vi "substreepbocht.vi"(4 "tijdsinterval 8":dbl, 5 "tijdsinterval 6":dbl, 6 "tijdsinterval 7":dbl, 7 "tijdsinterval in":dbl, 9 "tijdsinterval 5":dbl, 10 "tijdsinterval 3":dbl, 11 "tijdsinterval 4":dbl) -> ()   [LabVIEW 2019]
uses:
  <vilib>/myRIO/Common/Instrument Driver Framework/Utilities/typedefs/Analog Scaling Constants.ctl
  <vilib>/myRIO/Common/Instrument Driver Framework/Utilities/typedefs/Analog Scaling Constants List.ctl
  <vilib>/myRIO/Common/Instrument Driver Framework/myRIO v1.0/AO/typedefs/AO Channels Enum.ctl
  <vilib>/myRIO/Common/Instrument Driver Framework/myRIO v1.0/AO/typedefs/AO Channels List.ctl
  <vilib>/myRIO/Common/Instrument Driver Framework/Utilities/typedefs/Generic FPGA Reference.ctl
  <vilib>/myRIO/Common/Instrument Driver Framework/Utilities/typedefs/myRIO v1.0 Reference.ctl
  <vilib>/myRIO/Common/Instrument Driver Framework/Utilities/typedefs/Hardware Version Enum.ctl
  <vilib>/myRIO/Common/Instrument Driver Framework/Utilities/typedefs/myRIO Generic Hardware Reference.ctl
  <vilib>/myRIO/Instrument Drivers/Onboard IO/AO/typedefs/AO Reference.ctl
  <vilib>/myRIO/Instrument Drivers/Onboard IO/AO/AO.lvlib
  <vilib>/myRIO/Instrument Drivers/Onboard IO/AO/vis/Write.vi
  <vilib>/userDefined/High Color/nirio_resource_hc.ctl
  <vilib>/myRIO/Common/Instrument Driver Framework/myRIO v1.0/AO/vis/myRIO v1.1 Open AO.vi
  <vilib>/myRIO/Instrument Drivers/Onboard IO/AO/vis/myRIO AO Open.xnode
  <vilib>/myRIO/Common/Instrument Driver Framework/Utilities/vis/Is FPGA Ref Available.vi
  <vilib>/myRIO/Express VI/Onboard IO/AO/AO Express VI.xnode
  Global.vi
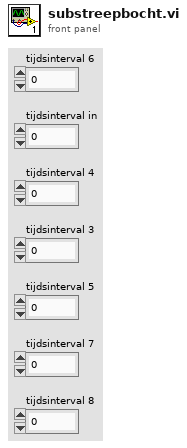
[diagram p1: front panel]
types:
  T1 = typedef "AO.lvlib/AO Reference.ctl" = cluster{"myRIO Reference":T2, "AO Channel List":T6, "AO Scaling Constant List":T8}
  T2 = typedef "myRIO Generic Hardware Reference.ctl" = cluster{"myRIO Model":T3, "myRIO Hardware Reference":T4}
  T3 = typedef "Hardware Version Enum.ctl" = enum16{"Unknown", "myRIO-1900", "myRIO-1950", "roboRIO", "NI ELVIS RIO CM", "ELVIS III"}
  T4 = typedef "myRIO v1.0 Reference.ctl" = cluster{"Generic FPGA Reference":T5, "Allow multiple opens":bool}
  T5 = typedef "Generic FPGA Reference.ctl" = refnum<k20>
  T6 = typedef "AO Channels List.ctl" = T7[]
  T7 = typedef "AO Channels Enum.ctl" = enum16{"Not Connected", "AudioOut/Left", "AudioOut/Right", "C/AO0", "C/AO1", "A/AO0", "A/AO1", "B/AO0", "B/AO1"}
  T8 = typedef "Analog Scaling Constants List.ctl" = T9[]
  T9 = typedef "Analog Scaling Constants.ctl" = cluster{"LSB Weight (Volts)":dbl, "Offset (Volts)":dbl, "Signed?":bool}
  T10 = typedef "nirio_resource_hc.ctl" = tag
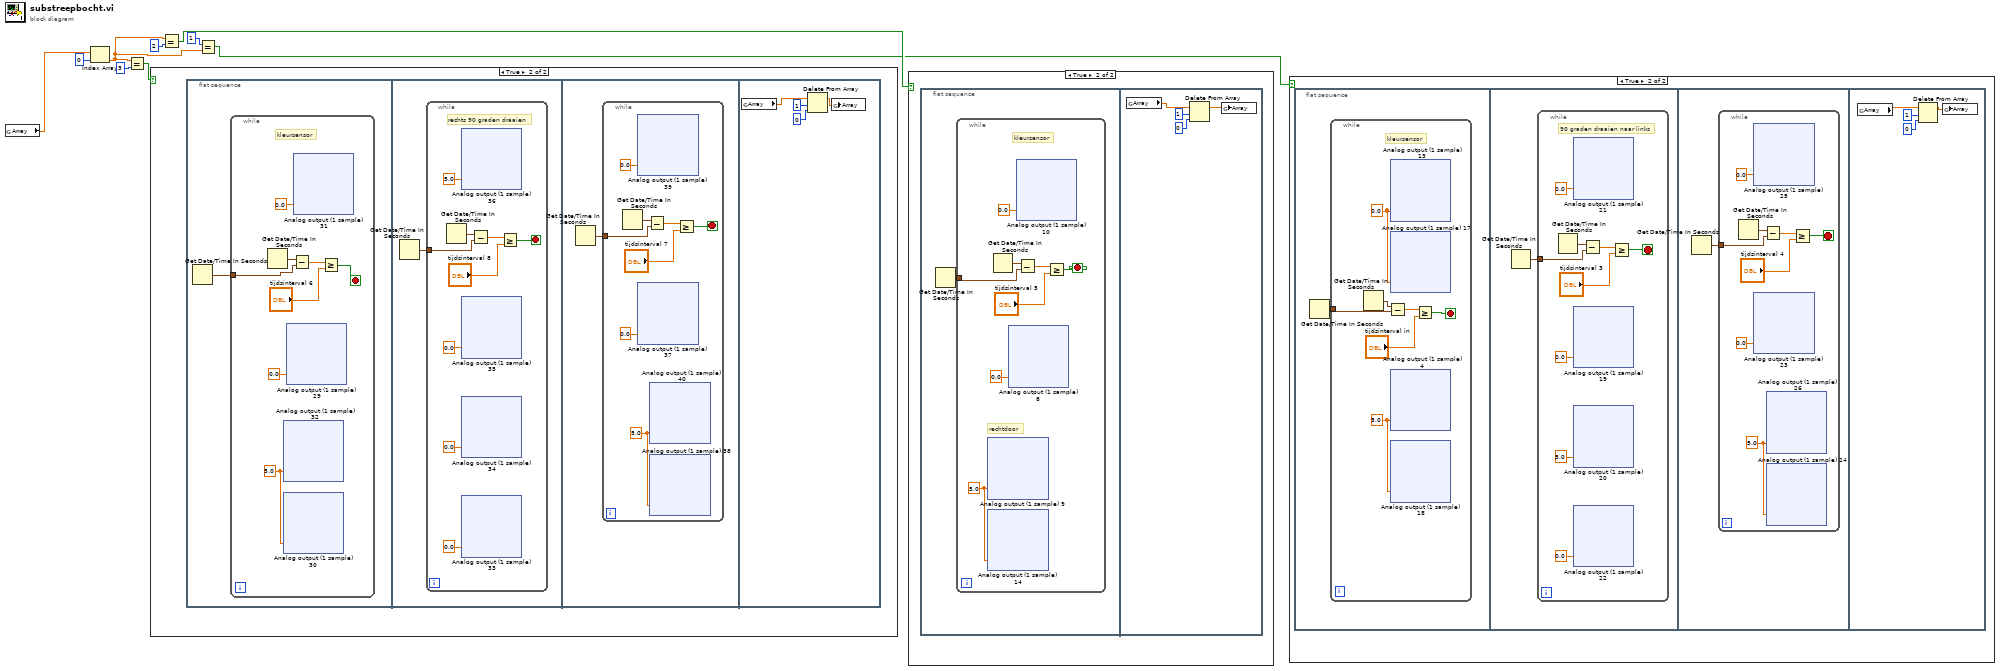
[diagram p0: block diagram]
diagram:
  n1 = global read "Global.vi" "Array"() -> (w9:dbl[])
  n2 = Index Array(array=w9, index=0) -> (element=w5:dbl)
  n3 = Equal?(x=w5, y=3) -> (x = y?=w3:bool)
  n4 = case shown="True" w3 {
    frame False {
    }
    frame True {
      n5 = flat-sequence {
        frame #0 {
          n6 = Get Date/Time In Seconds() -> (seconds since 1Jan1904=w10:timestamp)
          n7 = while {
            tunnel: w10 -> [w15]
            stop <- w11 stop-if-true
            w13 = 5.0
            # "kleursensor"
            n8 = Get Date/Time In Seconds() -> (seconds since 1Jan1904=w18:timestamp)
            n9 = xnode "Analog output (1 sample) 32"("A/AO0 (Pin 2)"=w13) -> ()  [unwired: 1 in, 1 out]
            n10 = xnode "Analog output (1 sample) 30"("B/AO0 (Pin 2)"=w13) -> ()  [unwired: 1 in, 1 out]
            n11 = xnode "Analog output (1 sample) 29"("B/AO1 (Pin 4)"=0.0) -> ()  [unwired: 1 in, 1 out]
            n12 = Subtract(x=w18, y=w15) -> (x-y=w16:dbl)
            n13 = xnode "Analog output (1 sample) 31"("A/AO1 (Pin 4)"=0.0) -> ()  [unwired: 1 in, 1 out]
            n14 = Greater Or Equal?(x=w16, y="tijdsinterval 6") -> (x >= y?=w11:bool)
          }
        }
        frame #1 {
          n15 = Get Date/Time In Seconds() -> (seconds since 1Jan1904=w167:timestamp)
          n16 = while {
            tunnel: w167 -> [w169]
            stop <- w170 stop-if-true
            # "rechts 90 graden draaien"
            n17 = Get Date/Time In Seconds() -> (seconds since 1Jan1904=w173:timestamp)
            n18 = xnode "Analog output (1 sample) 36"("A/AO0 (Pin 2)"=5.0) -> ()  [unwired: 1 in, 1 out]
            n19 = xnode "Analog output (1 sample) 35"("A/AO1 (Pin 4)"=0.0) -> ()  [unwired: 1 in, 1 out]
            n20 = xnode "Analog output (1 sample) 34"("B/AO0 (Pin 2)"=0.0) -> ()  [unwired: 1 in, 1 out]
            n21 = xnode "Analog output (1 sample) 33"("B/AO1 (Pin 4)"=0.0) -> ()  [unwired: 1 in, 1 out]
            n22 = Subtract(x=w173, y=w169) -> (x-y=w171:dbl)
            n23 = Greater Or Equal?(x=w171, y="tijdsinterval 8") -> (x >= y?=w170:bool)
          }
        }
        frame #2 {
          n24 = Get Date/Time In Seconds() -> (seconds since 1Jan1904=w325:timestamp)
          n25 = while {
            tunnel: w325 -> [w327]
            stop <- w326 stop-if-true
            w332 = 5.0
            n26 = Get Date/Time In Seconds() -> (seconds since 1Jan1904=w330:timestamp)
            n27 = xnode "Analog output (1 sample) 39"("A/AO1 (Pin 4)"=0.0) -> ()  [unwired: 1 in, 1 out]
            n28 = xnode "Analog output (1 sample) 37"("B/AO1 (Pin 4)"=0.0) -> ()  [unwired: 1 in, 1 out]
            n29 = Subtract(x=w330, y=w327) -> (x-y=w328:dbl)
            n30 = xnode "Analog output (1 sample) 40"("A/AO0 (Pin 2)"=w332) -> ()  [unwired: 1 in, 1 out]
            n31 = xnode "Analog output (1 sample) 38"("B/AO0 (Pin 2)"=w332) -> ()  [unwired: 1 in, 1 out]
            n32 = Greater Or Equal?(x=w328, y="tijdsinterval 7") -> (x >= y?=w326:bool)
          }
        }
        frame #3 {
          n33 = global read "Global.vi" "Array"() -> (w483:dbl[])
          n34 = Delete From Array(array=w483, length=1, index=0) -> (array with subset deleted=w482:dbl[])  [unwired: 1 out]
          n35 = global write "Global.vi" "Array"(w482) -> ()
        }
      }
    }
  }
  n36 = Equal?(x=w5, y=2) -> (x = y?=w2:bool)
  n37 = Equal?(x=1, y=w5) -> (x = y?=w1:bool)
  n38 = case shown="True" w2 {
    frame False {
    }
    frame True {
      n39 = flat-sequence {
        frame #0 {
          n40 = Get Date/Time In Seconds() -> (seconds since 1Jan1904=w486:timestamp)
          n41 = while {
            tunnel: w486 -> [w491]
            stop <- w487 stop-if-true
            w489 = 5.0
            # "rechtdoor"
            # "kleursensor"
            n42 = xnode "Analog output (1 sample) 9"("A/AO0 (Pin 2)"=w489) -> ()  [unwired: 1 in, 1 out]
            n43 = xnode "Analog output (1 sample) 14"("B/AO0 (Pin 2)"=w489) -> ()  [unwired: 1 in, 1 out]
            n44 = Get Date/Time In Seconds() -> (seconds since 1Jan1904=w492:timestamp)
            n45 = xnode "Analog output (1 sample) 8"("B/AO1 (Pin 4)"=0.0) -> ()  [unwired: 1 in, 1 out]
            n46 = xnode "Analog output (1 sample) 10"("A/AO1 (Pin 4)"=0.0) -> ()  [unwired: 1 in, 1 out]
            n47 = Subtract(x=w492, y=w491) -> (x-y=w494:dbl)
            n48 = Greater Or Equal?(x=w494, y="tijdsinterval 5") -> (x >= y?=w487:bool)
          }
        }
        frame #1 {
          n49 = global read "Global.vi" "Array"() -> (w644:dbl[])
          n50 = Delete From Array(array=w644, length=1, index=0) -> (array with subset deleted=w643:dbl[])  [unwired: 1 out]
          n51 = global write "Global.vi" "Array"(w643) -> ()
        }
      }
    }
  }
  n52 = case shown="True" w1 {
    frame False {
    }
    frame True {
      n53 = flat-sequence {
        frame #0 {
          n54 = Get Date/Time In Seconds() -> (seconds since 1Jan1904=w647:timestamp)
          n55 = while {
            tunnel: w647 -> [w651]
            stop <- w648 stop-if-true
            w650 = 0.0
            w649 = 5.0
            # "kleursensor"
            n56 = Get Date/Time In Seconds() -> (seconds since 1Jan1904=w652:timestamp)
            n57 = Subtract(x=w652, y=w651) -> (x-y=w654:dbl)
            n58 = xnode "Analog output (1 sample) 13"("A/AO1 (Pin 4)"=w650) -> ()  [unwired: 1 in, 1 out]
            n59 = xnode "Analog output (1 sample) 17"("B/AO1 (Pin 4)"=w650) -> ()  [unwired: 1 in, 1 out]
            n60 = xnode "Analog output (1 sample) 4"("A/AO0 (Pin 2)"=w649) -> ()  [unwired: 1 in, 1 out]
            n61 = xnode "Analog output (1 sample) 18"("B/AO0 (Pin 2)"=w649) -> ()  [unwired: 1 in, 1 out]
            n62 = Greater Or Equal?(x=w654, y="tijdsinterval in") -> (x >= y?=w648:bool)
          }
        }
        frame #1 {
          n63 = Get Date/Time In Seconds() -> (seconds since 1Jan1904=w803:timestamp)
          n64 = while {
            tunnel: w803 -> [w806]
            stop <- w805 stop-if-true
            # "90 graden draaien naar links"
            n65 = Get Date/Time In Seconds() -> (seconds since 1Jan1904=w809:timestamp)
            n66 = xnode "Analog output (1 sample) 21"("A/AO1 (Pin 4)"=0.0) -> ()  [unwired: 1 in, 1 out]
            n67 = xnode "Analog output (1 sample) 19"("B/AO1 (Pin 4)"=0.0) -> ()  [unwired: 1 in, 1 out]
            n68 = xnode "Analog output (1 sample) 20"("B/AO0 (Pin 2)"=5.0) -> ()  [unwired: 1 in, 1 out]
            n69 = xnode "Analog output (1 sample) 22"("A/AO0 (Pin 2)"=0.0) -> ()  [unwired: 1 in, 1 out]
            n70 = Subtract(x=w809, y=w806) -> (x-y=w807:dbl)
            n71 = Greater Or Equal?(x=w807, y="tijdsinterval 3") -> (x >= y?=w805:bool)
          }
        }
        frame #2 {
          n72 = Get Date/Time In Seconds() -> (seconds since 1Jan1904=w961:timestamp)
          n73 = while {
            tunnel: w961 -> [w963]
            stop <- w962 stop-if-true
            w968 = 5.0
            n74 = Get Date/Time In Seconds() -> (seconds since 1Jan1904=w966:timestamp)
            n75 = xnode "Analog output (1 sample) 25"("A/AO1 (Pin 4)"=0.0) -> ()  [unwired: 1 in, 1 out]
            n76 = xnode "Analog output (1 sample) 23"("B/AO1 (Pin 4)"=0.0) -> ()  [unwired: 1 in, 1 out]
            n77 = Subtract(x=w966, y=w963) -> (x-y=w964:dbl)
            n78 = xnode "Analog output (1 sample) 26"("A/AO0 (Pin 2)"=w968) -> ()  [unwired: 1 in, 1 out]
            n79 = xnode "Analog output (1 sample) 24"("B/AO0 (Pin 2)"=w968) -> ()  [unwired: 1 in, 1 out]
            n80 = Greater Or Equal?(x=w964, y="tijdsinterval 4") -> (x >= y?=w962:bool)
          }
        }
        frame #3 {
          n81 = global read "Global.vi" "Array"() -> (w1119:dbl[])
          n82 = Delete From Array(array=w1119, length=1, index=0) -> (array with subset deleted=w1118:dbl[])  [unwired: 1 out]
          n83 = global write "Global.vi" "Array"(w1118) -> ()
        }
      }
    }
  }
